vi "Test Helper Loop Broadcast Stopped State.vi"(8 "error in (no error)":errorcluster, 11 "Helper Loop Test In":refnum<class "Helper Loop Test.lvclass">) -> (0 "error out":errorcluster, 3 "Helper Loop Test Out":refnum<class "Helper Loop Test.lvclass">)   [LabVIEW 2020, in "Helper Loop Test.lvclass"]
uses:
  Helper Loop Test.lvclass
  C:/Program Files (x86)/National Instruments/LabVIEW 2020/vi.lib/Asteme/LUnit/Test Case.lvclass
  Mock Process/Mock Process.lvclass
  C:/Users/anton/Documents/GitHub/Triarc-Framework/source/Framework/Process/Process.lvclass
  <vilib>/Asteme/LUnit/Test Case.lvclass/Test Case.ctl
  <vilib>/Asteme/LUnit/LUnit Assertion Result.lvclass/LUnit Assertion Result.ctl
  Framework/Process/Process.lvclass/Process.ctl
  <vilib>/Asteme/LUnit/Palette/Pass If.vi
  <vilib>/Asteme/LUnit/Set Assertion Type.vi
  Support/Execution timer.vi
  Framework/Process/Private/SubVIs/Wait for finish.vi
  Framework/Process/Protected/Messaging/Enqueue Message.vi
  Framework/Process/Private/SubVIs/Set Lifecycle State.vi
  Framework/Process/Public/Lifecycle/Get Lifecycle State.vi
  <vilib>/Asteme/LUnit/Palette/Pass.vi
  <vilib>/Asteme/LUnit/Palette/Fail.vi
  <vilib>/Asteme/LUnit/Variant to string.vi
  <vilib>/Asteme/LUnit/LUnit Write Assertion Type.vi
  <vilib>/Utility/error.llb/Clear Errors.vi
  <vilib>/Asteme/LUnit/Add test result.vi
  <vilib>/Asteme/LUnit/LUnit Write Passed.vi
  <vilib>/Asteme/LUnit/LUnit Get Test Case.vi
  <vilib>/Asteme/LUnit/Assertion Result/LUnit Get Test Name.vi
  <vilib>/Asteme/LUnit/LUnit Write Message.vi
  <vilib>/Asteme/LUnit/LUnit Write Description.vi
  <vilib>/Asteme/LUnit/Read Test Case Name.vi
  Support/Event Helpers/Dequeue Event Message.vi
  <vilib>/Utility/error.llb/Error Cluster From Error Code.vi
  <vilib>/Utility/Data Type/Get Type Information.vi
  <vilib>/Utility/LVClass/Get LV Class Name.vi
  <vilib>/Asteme/LUnit/LUnit Assertion Result.lvclass
  Framework/Process/Process.lvclass
  <vilib>/Asteme/LUnit/Test Case.lvclass
  Support/Event Helpers/Event Helpers.lvlib
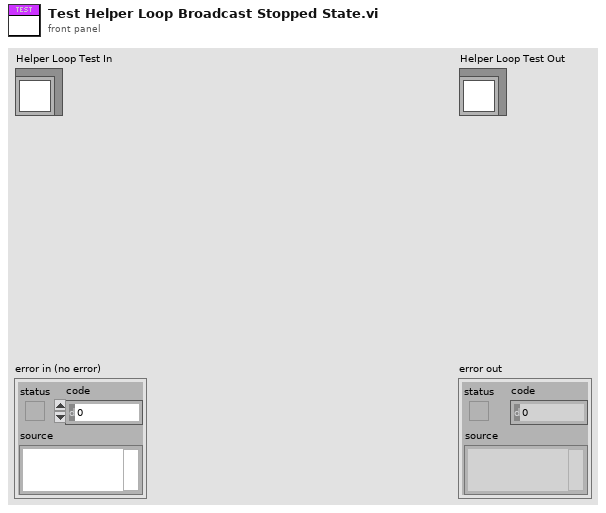
[diagram p1: front panel]
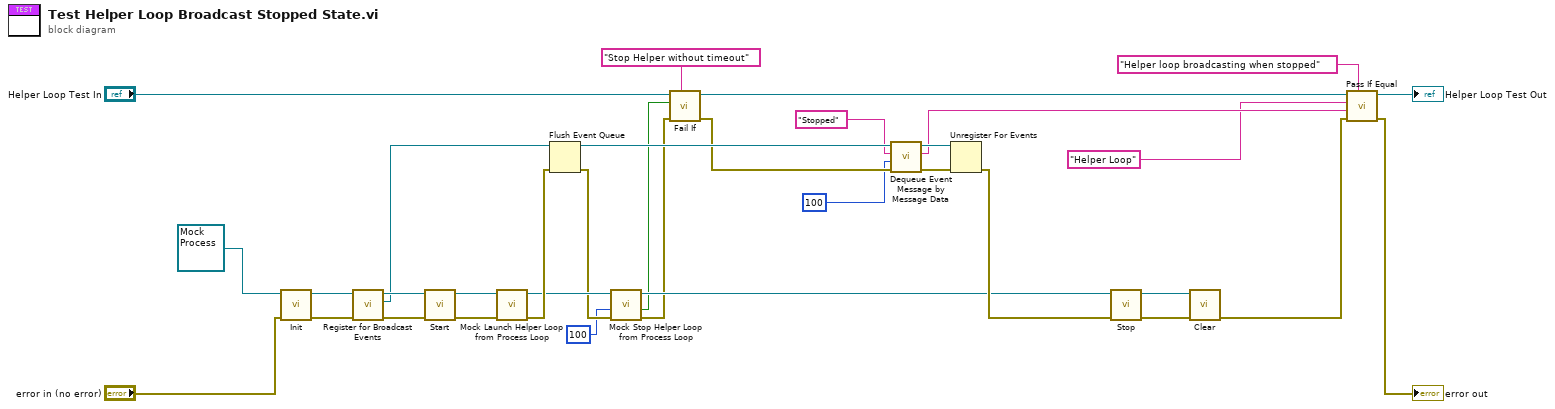
[diagram p0: block diagram]
diagram:
  n1 = call-dynamic "Init.vi"("error in (no error)"="error in (no error)", "Mock Process In"=refnum<class "Mock Process.lvclass"> refnum) -> ("error out"=w32:errorcluster, "Mock Process Out"=w33:refnum<class "Mock Process.lvclass">)  [unwired: 8 in]
  n2 = call "Register for Broadcast Events.vi"("error in (no error)"=w32, "Process In"=w33) -> ("error out"=w30:errorcluster, "Event Registration Refnum Out"=w20:refnum<event-registration>, "Process Out"=w31:refnum<class "Mock Process.lvclass">)  [unwired: 7 in]
  n3 = call "Start.vi"("error in (no error)"=w30, "Process In"=w31) -> ("error out"=w28:errorcluster, "Process Out"=w29:refnum<class "Mock Process.lvclass">)  [unwired: 8 in]
  n4 = call "Mock Launch Helper Loop from Process Loop.vi"("error in (no error)"=w28, "Mock Process in"=w29) -> ("error out"=w16:errorcluster, "Mock Process out"=w15:refnum<class "Mock Process.lvclass">)  [unwired: 8 in]
  n5 = Flush Event Queue(0:w20, 3:w16) -> (8:w17:refnum<event-registration>, 11:w13:errorcluster)  [unwired: 4 in, 1 out]
  n6 = call "Mock Stop Helper Loop from Process Loop.vi"("error in (no error)"=w13, "timeout in ms (-1)"=100, "Mock Process in"=w15) -> ("error out"=w10:errorcluster, "timed out?"=w8:bool, "Mock Process out"=w14:refnum<class "Mock Process.lvclass">)  [unwired: 6 in]
  n7 = call <vilib>:"Fail If.vi"("Description"="Stop Helper without timeout", "error in (no error)"=w10, "Fail?"=w8, "Test Case In"="Helper Loop Test In") -> ("error out"=w9:errorcluster, "Test Case Out"=w11:refnum<class "Helper Loop Test.lvclass">)  [unwired: 6 in]
  n8 = call "Dequeue Event Message by Message Data.vi"("error in (no error)"=w9, "Timeout (-1)"=100, "Message Data"="Stopped" ("y"), "Event Registration Refnum"=w17) -> ("error out"=w6:errorcluster, "Message"=w2:string, "Event Registration Refnum Out"=w19:refnum<event-registration>)  [unwired: 3 in, 2 out]
  n9 = Unregister For Events(event registration refnum=w19, error in=w6) -> (error out=w18:errorcluster)
  n10 = call "Stop.vi"("error in (no error)"=w18, "Process In"=w14) -> ("error out"=w27:errorcluster, "Process Out"=w3:refnum<class "Mock Process.lvclass">)  [unwired: 7 in, 1 out]
  n11 = call-dynamic "Clear.vi"("error in (no error)"=w27, "Mock Process In"=w3) -> ("error out"=w26:errorcluster)  [unwired: 9 in]
  n12 = call <vilib>:"Pass If Equal.vi"("Description"="Helper loop broadcasting when stopped", "error in (no error)"=w26, "Actual"=w2, "Expected"="Helper Loop" ("y"), "Test Case In"=w11) -> ("error out"=→"error out":errorcluster, "Test Case Out"=→"Helper Loop Test Out":refnum<class "Helper Loop Test.lvclass">)  [unwired: 5 in]
